vi "ForeBrainCommsTest.vi"() -> ()   [LabVIEW 2010]
uses:
  6-OCU Neurons/6.0-Super Heart Beat.ctl
  5-Forebrain/5.0-Global.vi
panel:
  out "4.7.4 - How UDP Client HB":T1
  out "4.7.4 - How UDP Client Error":errorcluster
  out "4.7.3 -What UDP Client HB":T1
  out "4.7.3 - What UDP Client Error":errorcluster
  out "4.7.2 - Where UDP Client HB":T1
  out "4.7.2 - Where UDP Client Error":errorcluster
  out "4.7.1 - Act UDP Server HB":T1
  out "4.7.1 - Act UDP Server Error":errorcluster
  in  "Stop Loops":bool
  in  "stop":bool
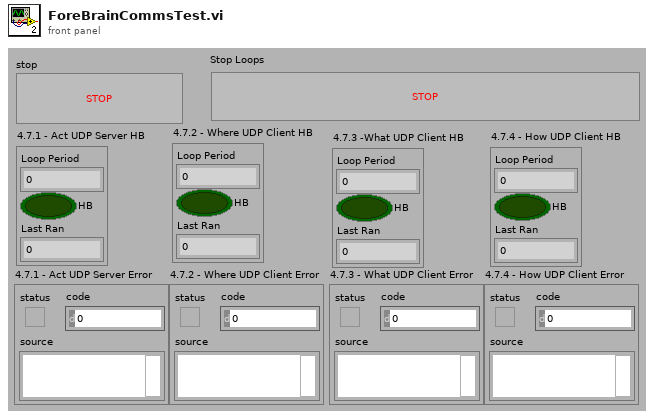
[diagram p1: front panel]
types:
  T1 = typedef "6.0-Super Heart Beat.ctl" = cluster{"Loop Period":u32, "HB":bool, "Last Ran":u32}
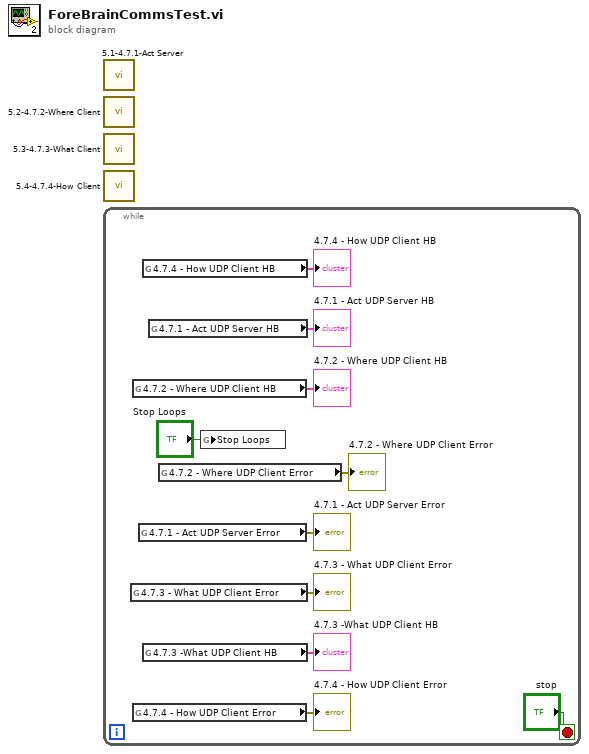
[diagram p0: block diagram]
diagram:
  n1 = call "5.1-4.7.1-Act Server.vi"() -> ()  [unwired: 1 in]
  n2 = call "5.2-4.7.2-Where Client.vi"() -> ()  [unwired: 7 in]
  n3 = call "5.3-4.7.3-What Client.vi"() -> ()  [unwired: 7 in]
  n4 = call "5.4-4.7.4-How Client.vi"() -> ()  [unwired: 7 in]
  n5 = while {
    stop <- "stop" stop-if-true
    n6 = global read "5.0-Global.vi" "4.7.3 - What UDP Client Error"() -> (→"4.7.3 - What UDP Client Error":errorcluster)
    n7 = global read "5.0-Global.vi" "4.7.2 - Where UDP Client HB"() -> (→"4.7.2 - Where UDP Client HB":T1)
    n8 = global read "5.0-Global.vi" "4.7.4 - How UDP Client Error"() -> (→"4.7.4 - How UDP Client Error":errorcluster)
    n9 = global read "5.0-Global.vi" "4.7.1 - Act UDP Server Error"() -> (→"4.7.1 - Act UDP Server Error":errorcluster)
    n10 = global read "5.0-Global.vi" "4.7.4 - How UDP Client HB"() -> (→"4.7.4 - How UDP Client HB":T1)
    n11 = global read "5.0-Global.vi" "4.7.3 -What UDP Client HB"() -> (→"4.7.3 -What UDP Client HB":T1)
    n12 = global read "5.0-Global.vi" "4.7.1 - Act UDP Server HB"() -> (→"4.7.1 - Act UDP Server HB":T1)
    n13 = global read "5.0-Global.vi" "4.7.2 - Where UDP Client Error"() -> (→"4.7.2 - Where UDP Client Error":errorcluster)
    n14 = global write "5.0-Global.vi" "Stop Loops"("Stop Loops") -> ()
  }
